vi "제목없음 2.vi"   [LabVIEW 2014]
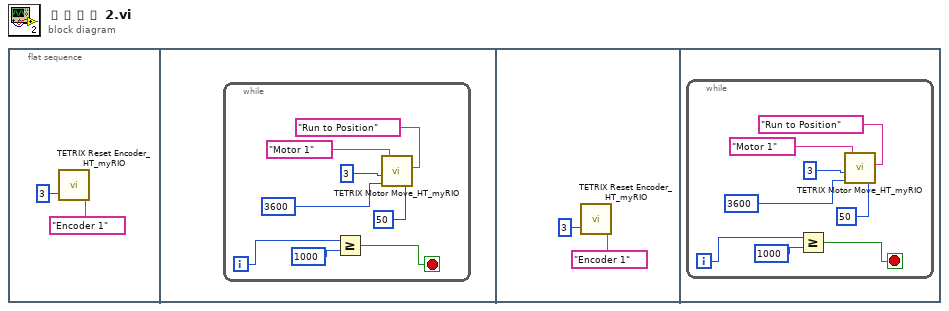
[diagram p0: block diagram]
diagram:
  n1 = flat-sequence {
    frame #0 {
      n2 = call <vilib>:"TETRIX Reset Encoder_HT_myRIO.vi"("Select Encoder"="Encoder 1", "Controller Daisy Chain Position ( 1 - 4)"=u8 3) -> ()  [unwired: 1 in, 1 out]
    }
    frame #1 {
      n3 = while {
        i -> [w6]
        stop <- w4 stop-if-true
        n4 = Greater Or Equal?(x=w6, y=1000) -> (x >= y?=w4:bool)
        n5 = call <vilib>:"TETRIX Motor Move_HT_myRIO.vi"("Power (-100 to 100)\n0 = Stop/Brake\n-128 = Stop/Coast"=i8 50 ("Motor 1 Power (-100 to 100)\n0 = Stop/Brake\n-128 = Stop/Coast"), "Control Mode"="Run to Position", "Encoder Target: 360 = 1 motor shaft revolution"=3600 ("Encoder 2 Target: 360 = 1 motor shaft revolution"), "Controller Daisy Chain Position: 1 - 4"=u8 3, "Select Channel"="Motor 1") -> ()  [unwired: 2 in, 1 out]
      }
    }
    frame #2 {
      n6 = call <vilib>:"TETRIX Reset Encoder_HT_myRIO.vi"("Select Encoder"="Encoder 1", "Controller Daisy Chain Position ( 1 - 4)"=u8 3) -> ()  [unwired: 1 in, 1 out]
    }
    frame #3 {
      n7 = while {
        i -> [w16]
        stop <- w14 stop-if-true
        n8 = Greater Or Equal?(x=w16, y=1000) -> (x >= y?=w14:bool)
        n9 = call <vilib>:"TETRIX Motor Move_HT_myRIO.vi"("Power (-100 to 100)\n0 = Stop/Brake\n-128 = Stop/Coast"=i8 50 ("Motor 1 Power (-100 to 100)\n0 = Stop/Brake\n-128 = Stop/Coast"), "Control Mode"="Run to Position", "Encoder Target: 360 = 1 motor shaft revolution"=3600 ("Encoder 2 Target: 360 = 1 motor shaft revolution"), "Controller Daisy Chain Position: 1 - 4"=u8 3, "Select Channel"="Motor 1") -> ()  [unwired: 2 in, 1 out]
      }
    }
  }
